vi "DMM_Set Reference.vi"(8 "error in (no error)":errorcluster, 10 "Instrument Reference":u8, 11 "DMM Virtual in":refnum<class "DMM Virtual.lvclass">) -> (0 "error out":errorcluster)   [LabVIEW 2018, in "DMM Virtual.lvclass"]
uses:
  DMM Virtual.lvclass
  DMM_Global.vi
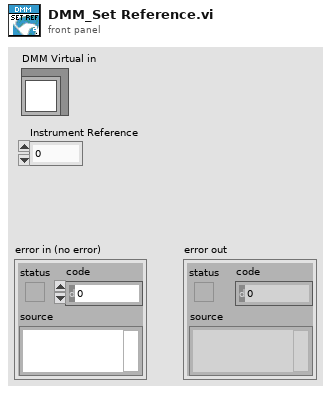
[diagram p1: front panel]
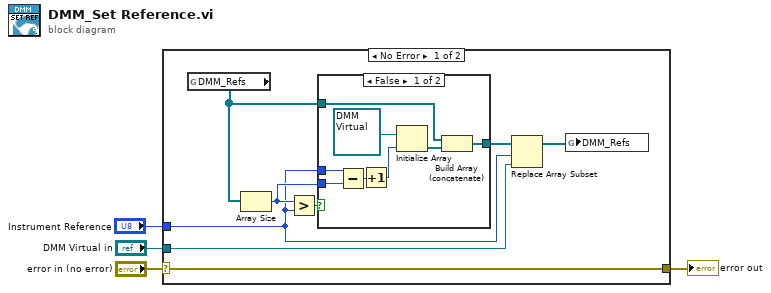
[diagram p0: block diagram]
diagram:
  n1 = case shown="No Error" "error in (no error)" {
    selector: "error in (no error)" -> [w7 w22]
    tunnel: "DMM Virtual in" -> [w9 _]
    tunnel: "Instrument Reference" -> [w8 _]
    tunnel: [w7 w22] -> w1
    frame No Error {
      n2 = global read "DMM_Global.vi" "DMM_Refs"() -> (w6:refnum<class "DMM Virtual.lvclass">[])
      n3 = Array Size(array=w6) -> (size(s)=w10:i32)
      n4 = Greater?(x=w10, y=w8) -> (0:w12:bool)
      n5 = case shown="False" w12 {
        tunnel: w8 -> [w19 _]
        tunnel: w6 -> [w20 w21]
        tunnel: w10 -> [w18 _]
        tunnel: [w15 w21] -> w11
        frame False {
          n6 = Subtract(x=w19, y=w18) -> (x-y=w17:i32)
          n7 = Increment(x=w17) -> (x+1=w16:i32)
          n8 = Initialize Array(refnum<class "DMM Virtual.lvclass"> refnum ("DMM Virtual.lvclass"), w16) -> (w14:refnum<class "DMM Virtual.lvclass">[])
          n9 = Build Array (concatenate)(w20, w14) -> (w15:refnum<class "DMM Virtual.lvclass">[])
        }
        frame True {
        }
      }
      n10 = Replace Array Subset(array=w11, new element=w9, index=w8) -> (w5:refnum<class "DMM Virtual.lvclass">[])
      n11 = global write "DMM_Global.vi" "DMM_Refs"(w5) -> ()
    }
    frame Error {
    }
  }
  "error out" <- w1
